vi "PutGetTreeNodeExpressionExample.vi"() -> ()   [LabVIEW 2010]
uses:
  <vilib>/builds/MDSplus/MDSplus/MDSplus.lvlib
panel:
  out "Expression  out":string=":NUM0"
  in  "Expression in":string=":NUM0"
  in  "Path":string=":NUM0"
  in  "Tree Shot":i32=-1
  in  "Tree Name":string="my_tree"
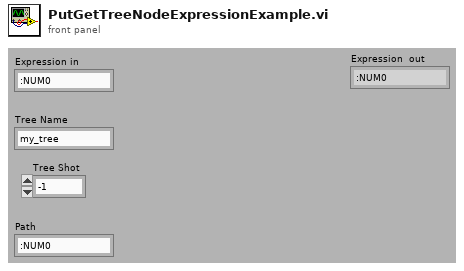
[diagram p1: front panel]
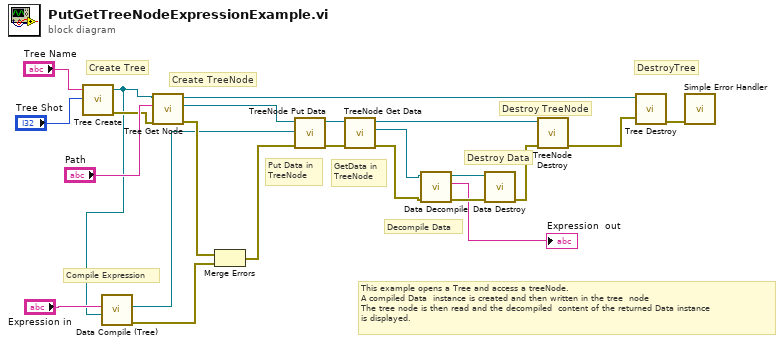
[diagram p0: block diagram]
diagram:
  # "This example opens a Tree and access a treeNode.\nA compiled Data  instance is created and then written in the tree  node\nThe tree node is then read and the decompiled  content of the returned Data instance\nis displayed."
  # "DestroyTree"
  # "Destroy TreeNode"
  # "Destroy Data"
  # "Decompile Data"
  # "GetData in\nTreeNode"
  # "Put Data in\nTreeNode"
  # "Compile Expression"
  # "Create TreeNode"
  # "Create Tree"
  n1 = call <vilib>:"Tree Create.vi"("Shot"="Tree Shot", "Name"="Tree Name") -> ("error out"=w12:errorcluster, "Tree DVR out"=w3:refnum<data-value>)  [unwired: 8 in]
  n2 = call <vilib>:"Data Compile (Tree).vi"("Tree in"=w3, "Expression"="Expression in") -> ("error out"=w1:errorcluster, "Data out"=w2:refnum<data-value>)  [unwired: 6 in, 2 out]
  n3 = call <vilib>:"Tree Get Node.vi"("error in (no error)"=w12, "Path"="Path", "Tree DVR in"=w3) -> ("error out"=w16:errorcluster, "Node out"=w17:refnum<data-value>, "Tree DVR out"=w11:refnum<data-value>)  [unwired: 6 in]
  n4 = Merge Errors(w16, w1) -> (w22:errorcluster)
  n5 = call <vilib>:"TreeNode Put Data.vi"("error in (no error)"=w22, "Data"=w2, "TreeNode DVR in"=w17) -> ("error out"=w20:errorcluster, "TreeNode DVR out"=w21:refnum<data-value>)  [unwired: 7 in]
  n6 = call <vilib>:"TreeNode Get Data.vi"("error in (no error)"=w20, "TreeNode DVR in"=w21) -> ("error out"=w7:errorcluster, "Data out"=w8:refnum<data-value>, "TreeNode DVR out"=w10:refnum<data-value>)  [unwired: 7 in]
  n7 = call <vilib>:"Data Decompile.vi"("error in (no error)"=w7, "Data DVR in"=w8) -> ("error out"=w6:errorcluster, "Expression out"=→"Expression  out":string, "Data DVR out"=w5:refnum<data-value>)  [unwired: 7 in]
  n8 = call <vilib>:"Data Destroy.vi"("error in (no error)"=w6, "Data DVR in"=w5) -> ("error out"=w19:errorcluster)  [unwired: 9 in]
  n9 = call <vilib>:"TreeNode Destroy.vi"("error in (no error)"=w19, "TreeNode DVR in"=w10) -> ("error out"=w15:errorcluster)  [unwired: 9 in]
  n10 = call <vilib>:"Tree Destroy.vi"("error in (no error)"=w15, "Tree DVR in"=w11) -> ("error out"=w18:errorcluster)  [unwired: 9 in]
  n11 = call <vilib>:"Simple Error Handler.vi"("error in (no error)"=w18) -> ()  [unwired: 4 in, 5 out]
